vi "Update Set-Points From Last Recording.vi"   [LabVIEW 2013]
uses:
  <vilib>/Analysis/baseanly.llb/Mean (DBL).vi
  <vilib>/Analysis/NI_AALBase.lvlib
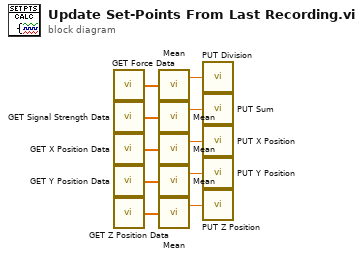
[diagram p0: block diagram]
diagram:
  n1 = call "GET Force Data.vi"() -> ("Force Data"=w5:dbl[])
  n2 = call "GET Signal Strength Data.vi"() -> ("Signal Strength Data"=w4:dbl[])
  n3 = call "GET X Position Data.vi"() -> ("X Position Data"=w3:dbl[])
  n4 = call "GET Y Position Data.vi"() -> ("Y Position Data"=w2:dbl[])
  n5 = call "GET Z Position Data.vi"() -> ("Z Position Data"=w1:dbl[])
  n6 = call-poly <vilib>:"Mean.vi"("X"=w5) -> ("mean"=w7:dbl)  [unwired: 1 out]
  n7 = call-poly <vilib>:"Mean.vi"("X"=w4) -> ("mean"=w8:dbl)  [unwired: 1 out]
  n8 = call-poly <vilib>:"Mean.vi"("X"=w3) -> ("mean"=w9:dbl)  [unwired: 1 out]
  n9 = call-poly <vilib>:"Mean.vi"("X"=w2) -> ("mean"=w10:dbl)  [unwired: 1 out]
  n10 = call-poly <vilib>:"Mean.vi"("X"=w1) -> ("mean"=w6:dbl)  [unwired: 1 out]
  n11 = call "PUT Division.vi"("Division"=w7) -> ()
  n12 = call "PUT Sum.vi"("Sum"=w8) -> ()
  n13 = call "PUT X Position.vi"("X Position"=w9) -> ()
  n14 = call "PUT Y Position.vi"("Y Position"=w10) -> ()
  n15 = call "PUT Z Position.vi"("Z Position"=w6) -> ()
